vi "GUI_NDCXIIGlassman.vi"() -> ()   [LabVIEW 2013]
uses:
  Shared/GUI_Template/GUI_master/tcp_new_data_event.ctl
  Shared/GUI_Template/GUI_master/tcp new data cluster.ctl
panel:
  in  "reading.channel 3::6":enum16{"on", "off"}(ring) caption="reading.channel 1::6"
  in  "reading.channel 1::6":enum16{"on", "off"}(ring)
  in  "reading.channel 2::6":enum16{"on", "off"}(ring) caption="reading.channel 1::6"
  in  "reading.channel 1::10":enum16{"on", "off"}(ring) caption="reading.channel 1::6"
  in  "reading.channel 2::10":enum16{"on", "off"}(ring) caption="reading.channel 1::6"
  in  "reading.channel 1::11":enum16{"on", "off"}(ring) caption="reading.channel 1::6"
  in  "reading.channel 2::11":enum16{"on", "off"}(ring) caption="reading.channel 1::6"
  in  "reading.channel 1::9":enum16{"on", "off"}(ring) caption="reading.channel 1::6"
  in  "reading.channel 2::9":enum16{"on", "off"}(ring) caption="reading.channel 1::6"
  in  "reading.channel 1::8":enum16{"on", "off"}(ring) caption="reading.channel 1::6"
  in  "reading.channel 2::8":enum16{"on", "off"}(ring) caption="reading.channel 1::6"
  in  "reading.channel 2::7":enum16{"on", "off"}(ring) caption="reading.channel 1::6"
  in  "HV5 enable":bool=TRUE
  in  "HV4 enable":bool=TRUE
  in  "HV3 enable":bool=TRUE
  in  "HV2 enable":bool=TRUE
  in  "HV1 enable":bool=TRUE
  in  "GUIdevice 11":string="GlassMan-Basement5-enable" caption="GUIdevice 6"
  in  "GUIdevice 10":string="GlassMan-Basement4-enable" caption="GUIdevice 6"
  in  "GUIdevice 9":string="GlassMan-Basement3-enable" caption="GUIdevice 6"
  in  "GUIdevice 8":string="GlassMan-Basement2-enable" caption="GUIdevice 6"
  in  "GUIdevice 7":string="GlassMan-Basement1-enable" caption="GUIdevice 6"
  in  "reading.channel 1::7":enum16{"on", "off"}(ring) caption="reading.channel 1::6"
  in  "all on":bool=TRUE caption="Rack AC ON"
  in  "GUIdevice 6":string="BasementRackPower"
  in  "GUIdevice 5":string="GlassMan-Basement5"
  in  "GUIdevice 4":string="GlassMan-Basement4"
  in  "GUIdevice 3":string="GlassMan-Basement3"
  in  "voltage::5":dbl caption="Voltage from GM5" min=0.0 max=10.0
  out "current::5":dbl caption="Current from GM5" min=0.0 max=5.0
  in  "voltage::4":dbl caption="Voltage from GM4" min=0.0 max=10.0
  out "current::4":dbl caption="Current from GM4" min=0.0 max=5.0
  in  "voltage::3":dbl caption="Voltage from Voltage from GM3" min=0.0 max=10.0
  out "current::3":dbl caption="Current from GM3" min=0.0 max=5.0
  in  "voltage::2":dbl caption="Voltage from GM2" min=0.0 max=10.0
  out "current::2":dbl caption="Current from GM2" min=0.0 max=5.0
  in  "GUIdevice 2":string="GlassMan-Basement2"
  out "current::1":dbl caption="Current from GM1" min=0.0 max=5.0
  in  "voltage::1":dbl caption="Voltage from GM1" min=0.0 max=10.0
  in  "stop":bool
  in  "GUIdevice 1":string="GlassMan-Basement1"
  out "tcp data event":T1
  out "error IO 2":errorcluster
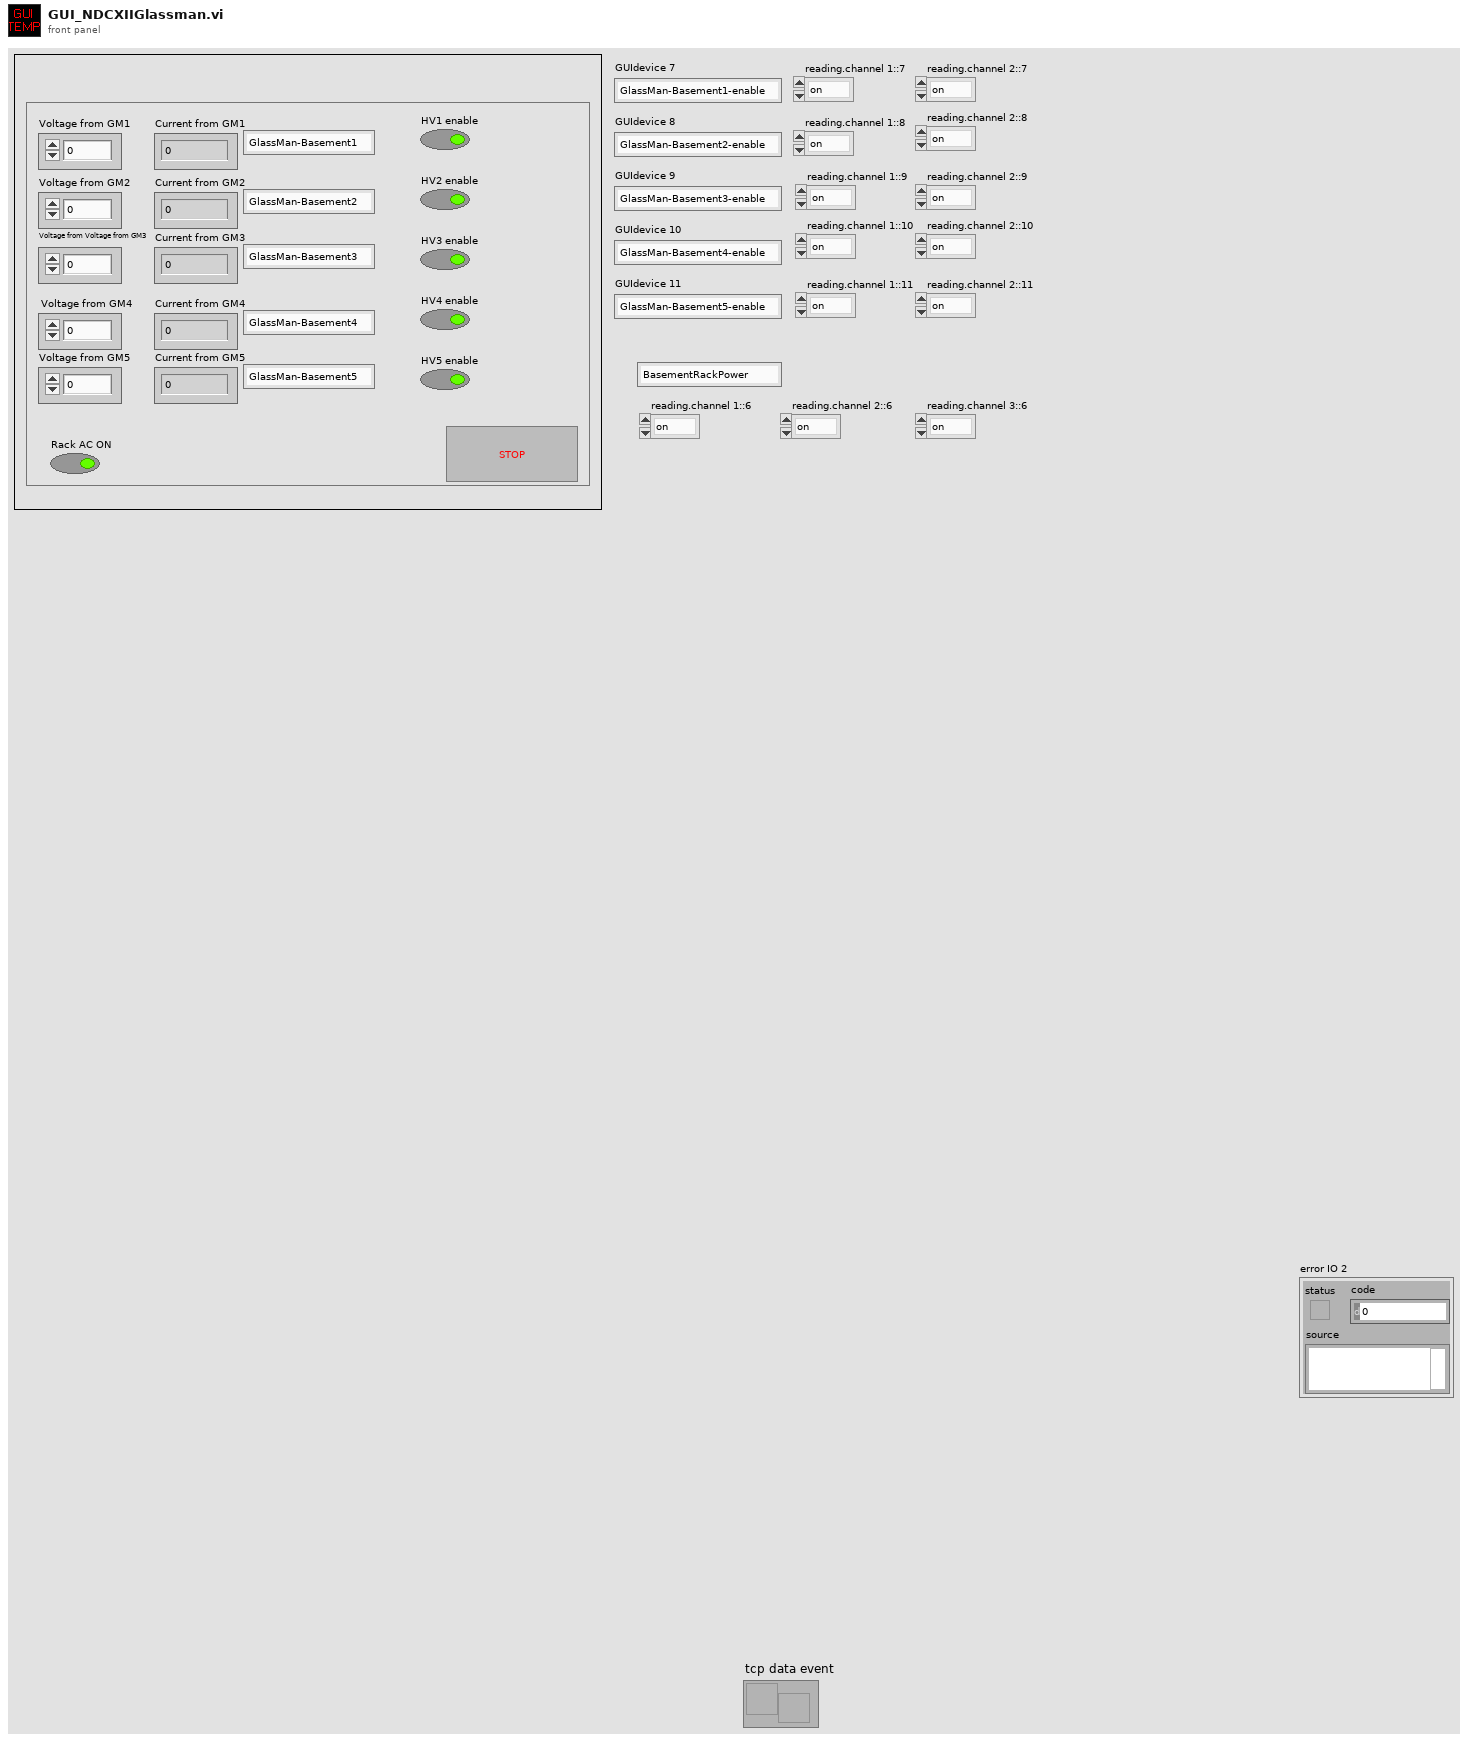
[diagram p1: front panel]
types:
  T1 = typedef "tcp_new_data_event.ctl" = refnum<user-event>
  T2 = typedef "tcp new data cluster.ctl" = cluster{"EventEnum":enum16{"new data", "connection status update"}, "Device name":string}
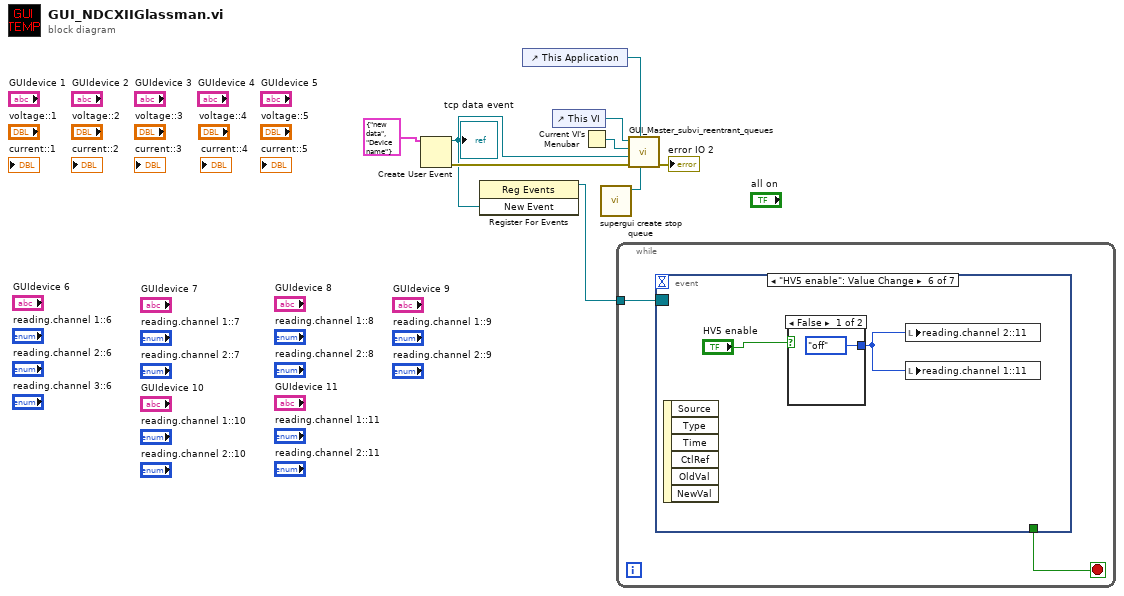
[diagram p0: block diagram]
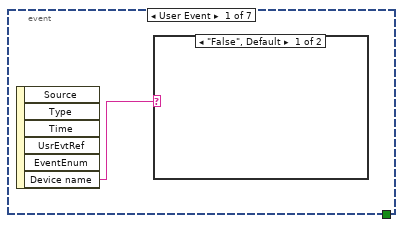
[diagram p2: hidden frame]
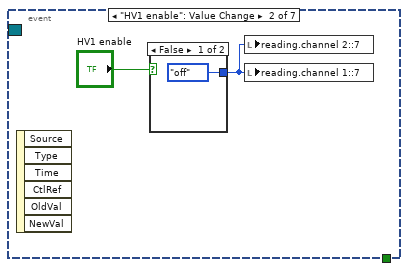
[diagram p4: hidden frame]
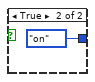
[diagram p5: hidden frame]
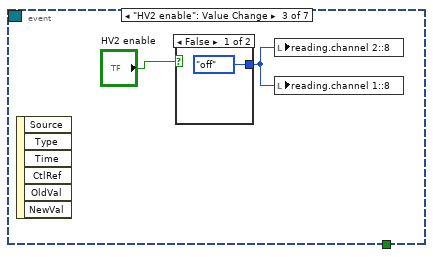
[diagram p6: hidden frame]
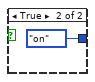
[diagram p7: hidden frame]
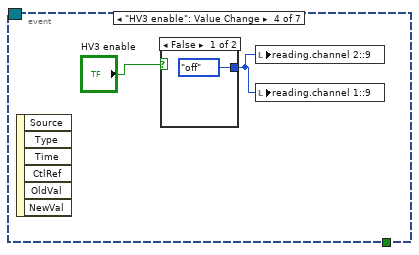
[diagram p8: hidden frame]
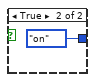
[diagram p9: hidden frame]
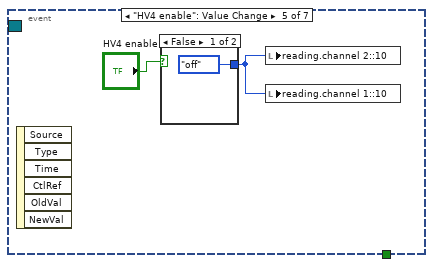
[diagram p10: hidden frame]
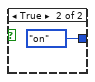
[diagram p11: hidden frame]
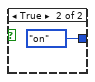
[diagram p12: hidden frame]
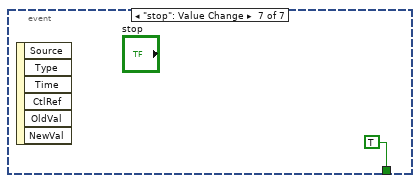
[diagram p13: hidden frame]
diagram:
  n1 = Create User Event(user event datatype=T2 {"EventEnum"=enum."new data", "Device name"="Device name"} ("New Event")) -> (user event=w4:refnum<user-event>, error out=w5:errorcluster)  [unwired: 1 in]
  "tcp data event" <- w4
  n2 = register-events(w4) -> (reference out=w2:refnum<event-registration>)  [unwired: 2 in, 1 out]
  n3 = control-ref of="This Application"() -> (w3:refnum<vi>)
  n4 = control-ref of="This VI"() -> (w8:refnum<vi>)
  n5 = Current VI's Menubar() -> (w7:refnum<k9>)
  n6 = call "supergui create stop queue.vi"() -> ("STOP Queue out"=w1:refnum<queue>)  [unwired: 11 in]
  n7 = while {
    tunnel: w2 -> [w11]
    stop <- w10 stop-if-true
    n8 = event shown="[5] \"HV5 enable\": Value Change" {
      selector: w11 -> [_ _ _ _ _ _ _]
      dyn-events: _ -> [_ _ _ _ _ _ _]
      timeout: _ -> [_ _ _ _ _ _ _]
      tunnel: [_ _ _ _ _ _ TRUE ("stop")] -> w10
      event User Event {
        n9 = event-data() -> ("Device name"=w12:string)  [unwired: 1 in, 5 out]
        n10 = case shown="\"False\", Default" w12 {
          frame "False", Default {
          }
          frame "Basement-Glassman1" {
          }
        }
      }
      event "HV1 enable": Value Change {
        n11 = event-data() -> ()  [unwired: 1 in, 6 out]
        n12 = case shown="False" "HV1 enable" {
          tunnel: [enum16{"on", "off"}."off" ("reading.channel 2::7") enum16{"on", "off"}."on" ("reading.channel 2::7")] -> w13
          frame False {
          }
          frame True {
          }
        }
        n13 = local write "reading.channel 2::7"(w13) -> ()
        n14 = local write "reading.channel 1::7"(w13) -> ()
      }
      event "HV2 enable": Value Change {
        n15 = event-data() -> ()  [unwired: 1 in, 6 out]
        n16 = case shown="False" "HV2 enable" {
          tunnel: [enum16{"on", "off"}."off" ("reading.channel 2::7") enum16{"on", "off"}."on" ("reading.channel 2::7")] -> w17
          frame False {
          }
          frame True {
          }
        }
        n17 = local write "reading.channel 2::8"(w17) -> ()
        n18 = local write "reading.channel 1::8"(w17) -> ()
      }
      event "HV3 enable": Value Change {
        n19 = event-data() -> ()  [unwired: 1 in, 6 out]
        n20 = case shown="False" "HV3 enable" {
          tunnel: [enum16{"on", "off"}."off" ("reading.channel 2::7") enum16{"on", "off"}."on" ("reading.channel 2::7")] -> w21
          frame False {
          }
          frame True {
          }
        }
        n21 = local write "reading.channel 2::9"(w21) -> ()
        n22 = local write "reading.channel 1::9"(w21) -> ()
      }
      event "HV4 enable": Value Change {
        n23 = event-data() -> ()  [unwired: 1 in, 6 out]
        n24 = case shown="False" "HV4 enable" {
          tunnel: [enum16{"on", "off"}."off" ("reading.channel 2::7") enum16{"on", "off"}."on" ("reading.channel 2::7")] -> w25
          frame False {
          }
          frame True {
          }
        }
        n25 = local write "reading.channel 2::10"(w25) -> ()
        n26 = local write "reading.channel 1::10"(w25) -> ()
      }
      event "HV5 enable": Value Change {
        n27 = event-data() -> ()  [unwired: 1 in, 6 out]
        n28 = case shown="False" "HV5 enable" {
          tunnel: [enum16{"on", "off"}."off" ("reading.channel 2::7") enum16{"on", "off"}."on" ("reading.channel 2::7")] -> w29
          frame False {
          }
          frame True {
          }
        }
        n29 = local write "reading.channel 2::11"(w29) -> ()
        n30 = local write "reading.channel 1::11"(w29) -> ()
      }
      event "stop": Value Change {
        n31 = event-data() -> ()  [unwired: 1 in, 6 out]
      }
    }
  }
  n32 = call "GUI_Master_subvi_reentrant_queues.vi"("STOP Queue in"=w1, "This Application"=w3, "error in (no error)"=w5, "tcp data event"=w4, "Caller menu reference"=w7, "Caller VI ref"=w8) -> ("error out"=→"error IO 2":errorcluster)  [unwired: 5 in]
